vi "SDL Renderer Clear.vi"(11 "Main Controller Actor":refnum<class "Main Controller Actor.lvclass">) -> ()   [LabVIEW 2021, in "Main Controller Actor.lvclass"]
uses:
  Main Controller Actor.lvclass
  Main Controller Actor.lvclass/Main Controller Actor.ctl
  LabSDL2/Source/Libraries/LibSDL2 Wrapper/LibSDL2.lvlib
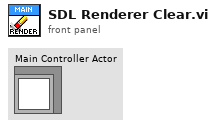
[diagram p1: front panel]
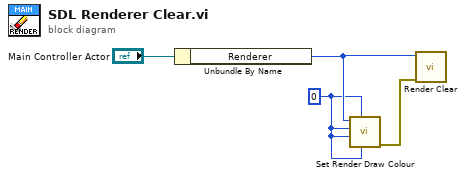
[diagram p0: block diagram]
diagram:
  w2 = u8 0 ("A")
  n1 = Unbundle By Name("Main Controller Actor") -> ("Renderer"=w4:u32)
  n2 = call "Set Render Draw Colour.vi"("B"=w2, "A"=w2, "G"=w2, "R"=w2, "Renderer Pointer"=w4) -> ("error out"=w3:errorcluster)  [unwired: 5 in, 1 out]
  n3 = call "Render Clear.vi"("error in"=w3, "Renderer Pointer"=w4) -> ()  [unwired: 8 in, 2 out]
